vi "Compute Pseudo UC Wrapper.vi"(8 "error in (no error)":errorcluster, 11 "VI in":refnum<vi>) -> (0 "error out":errorcluster, 2 "Notebook String":string, 3 "Plot Name":string)   [LabVIEW 2019]
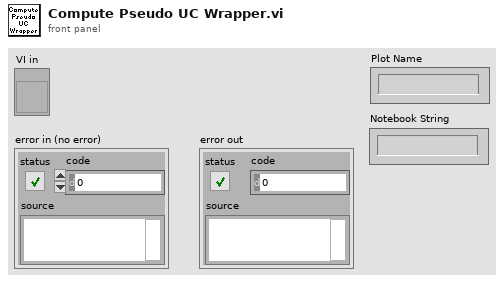
[diagram p1: front panel]
types:
  T1 = typedef "Pseudo Phasor Parameters.ctl" = cluster{"Display Parameters":T2, "Phasor Parameters":T4, "Decay & IRF Parameters":T7, "Gate Parameters":T9, "Detector Parameters":T11}
  T2 = typedef "Phasor Explorer Display Parameters.ctl" = cluster{"# Points":i32, "Ramp Type":enum16{"Linear", "Logarithmic"}, "Type of Series":T3, "Min tau":dbl[unit], "Max tau":dbl[unit], "Include 0":bool, "Include Infinity":bool}
  T3 = typedef "Type of Series.ctl" = enum16{"1-Exp Decays", "Linear Combination of 1-Exp"}
  T4 = typedef "Phasor Explorer Phasor Parameters.ctl" = cluster{"Harmonic frequency":dbl[unit], "Use f* = 1/D Frequency":bool, "Calibrated Phasor":bool, "Calibration Lifetime":dbl[unit], "Phasor Calculation":T5, "SEPL Type":T6, "# Gates":dbl, "Square Gate Width":dbl[unit], "Show Ticks":bool}
  T5 = typedef "Phasor Calculation Type.ctl" = enum16{"Direct Sum", "Analytical Formula"}
  T6 = typedef "Phasor Type.ctl" = enum16{"UC", "L_N", "L_N[W]"}
  T7 = typedef "Phasor Explorer Decay Parameters.ctl" = cluster{"Lifetime":dbl[unit], "IRF Offset":dbl[unit], "Laser Period":dbl[unit], "Normalized Decays":bool, "IRF Model":T8, "IRF Parameter 1":dbl[unit]}
  T8 = typedef "IRF Model.ctl" = enum16{"Dirac", "Exponential"}
  T9 = typedef "Phasor Explorer Gate Parameters.ctl" = cluster{"First Gate Start":dbl[unit], "Use Gate Center":bool, "Gate Width":dbl[unit], "Gate Step":dbl[unit], "# Gates":dbl, "Gate Type":T10, "Edge Width":dbl[unit], "Top Slope":dbl[unit], "Reversed Sawtooth?":bool, "Analytical Computation":bool, "Tolerance":dbl, "Integration":enum32{"Item 0", "Item 1"}, "# Steps":dbl, "Type of User-defined Function":enum32{"Gate", "IRF"}}
  T10 = typedef "Gate Type.ctl" = enum16{"Square", "Finite Edge Square", "Finite Edge, Tilted Top Square", "Triangle", "Sawtooth", "User-defined"}
  T11 = typedef "Phasor Explorer Detector Parameters.ctl" = cluster{"Frames/Image":i32, "Gates/Frame":i32, "Bits/Frame":i32, "Multiplicity":i32, "Incident Signal":dbl}
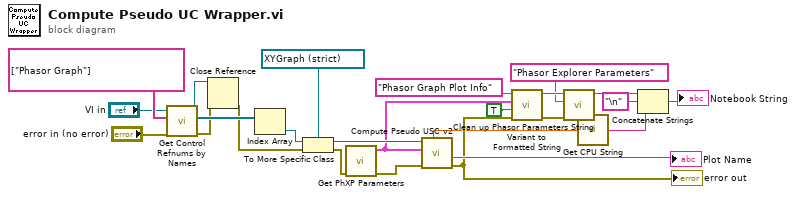
[diagram p0: block diagram]
diagram:
  n1 = call "Get Control Refnums by Names.vi"("error in"="error in (no error)", "Control Labels"=string[] ["Phasor Graph"], "VI  Ref"="VI in") -> ("error out"=w6:errorcluster, "Ctl Refnums"=w21:refnum<vi>[], "VI  Ref (out)"=w22:refnum<vi>)  [unwired: 5 in, 1 out]
  n2 = Close Reference(reference=w22, error in (no error)=w6) -> (error out=w5:errorcluster)
  n3 = Index Array(array=w21) -> (element=w19:refnum<vi>)  [unwired: 1 in]
  n4 = To More Specific Class(target class=refnum<vi> refnum ("Phasor Graph Refnum"), reference=w19, error in=w5) -> (specific class reference=w18:refnum<vi>, error out=w16:errorcluster)
  n5 = call "Get PhXP Parameters.vi"("Error In"=w16) -> ("Error Out"=w15:errorcluster, "Phasor Explorer Parameters"=w9:T1)  [unwired: 7 in, 2 out]
  n6 = call "Compute Pseudo USC v2.vi"("Error In"=w15, "Phasor Parameters"=w9, "Phasor Graph Refnum"=w18) -> ("Error Out"=w8:errorcluster, "Plot Name"=→"Plot Name":string, "CPU (s)"=w4:dbl)  [unwired: 3 in, 3 out]
  "error out" <- w8
  n7 = call "Variant to Formatted String.vi"("Error In"=w8, "Hide Long Cluster Names (T)"=TRUE ("Hide Long Names (Cluster)"), "Variant"=w9, "Label"="Phasor Graph Plot Info") -> ("Error Out"=w11:errorcluster, "String"=w12:string)  [unwired: 6 in]
  n8 = call "Clean up Phasor Parameters String.vi"("Error In"=w11, "Cluster Label"="Phasor Explorer Parameters" ("regular expression"), "String in"=w12) -> ("String out"=w7:string)  [unwired: 7 in, 1 out]
  n9 = call "Get CPU String.vi"("CPU (s)"=w4) -> ("String"=w2:string)  [unwired: 8 in]
  n10 = Concatenate Strings(w7, "\n" ("string"), w2) -> (→"Notebook String":string)
